vi "SensorLabview.vi"() -> ()   [LabVIEW 2020]
panel:
  in  "Water Pipe Ready":bool
  in  "Plant Health":string
  in  "Weed Detected":string
  out "VISA Error":string
  out "Return Count":dbl
  out "Website Status":string
  out "Command Status":string
  out "Pump Done Message":string
  out "Pump Command":string
  out "PumpCode":dbl
  out "Pump Duration":dbl
  out "Humidity Snapshot":dbl
  out "Temperature Snapshot":dbl
  out "Moisture %":dbl
  out "Current Pot Number":dbl
  out "Live Temperature °C":dbl
  out "Live Humidity %":dbl
  out "Selected Moisture %":dbl
  out "Humidity Voltage":dbl
  out "LM35 Voltage":dbl
  out "Selected Soil Voltage":dbl
  in  "Number of Pots":dbl
  in  "Max Pump Time":dbl
  in  "K Value":dbl
  in  "Target Moisture":dbl
  in  "Hhigh":dbl
  in  "Hlow":dbl
  in  "Vwet":dbl
  in  "Vdry":dbl
  in  "stop":bool
  in  "Robot Stop Detected":bool
  in  "ESP32 COM Port":refnum<visa-resource-name>
  # "Live Sensor Indicators"
  # "Calibration controls"
  # "System Controls"
  # "Pot snapshot indicators"
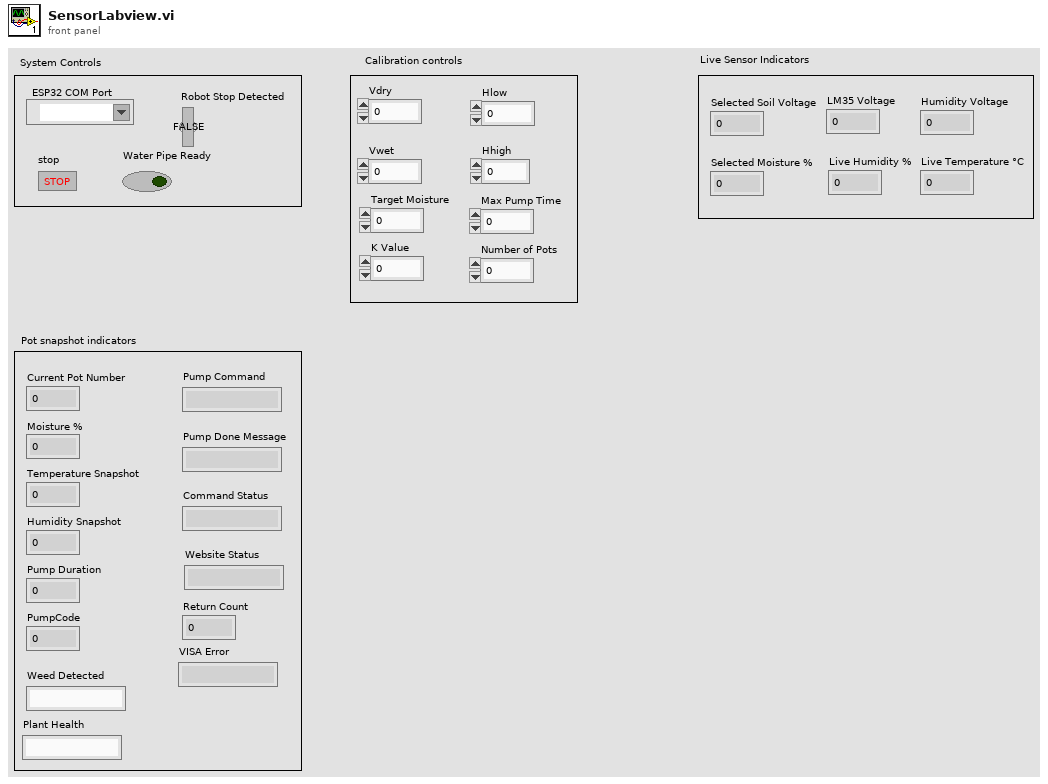
[diagram p1: front panel]
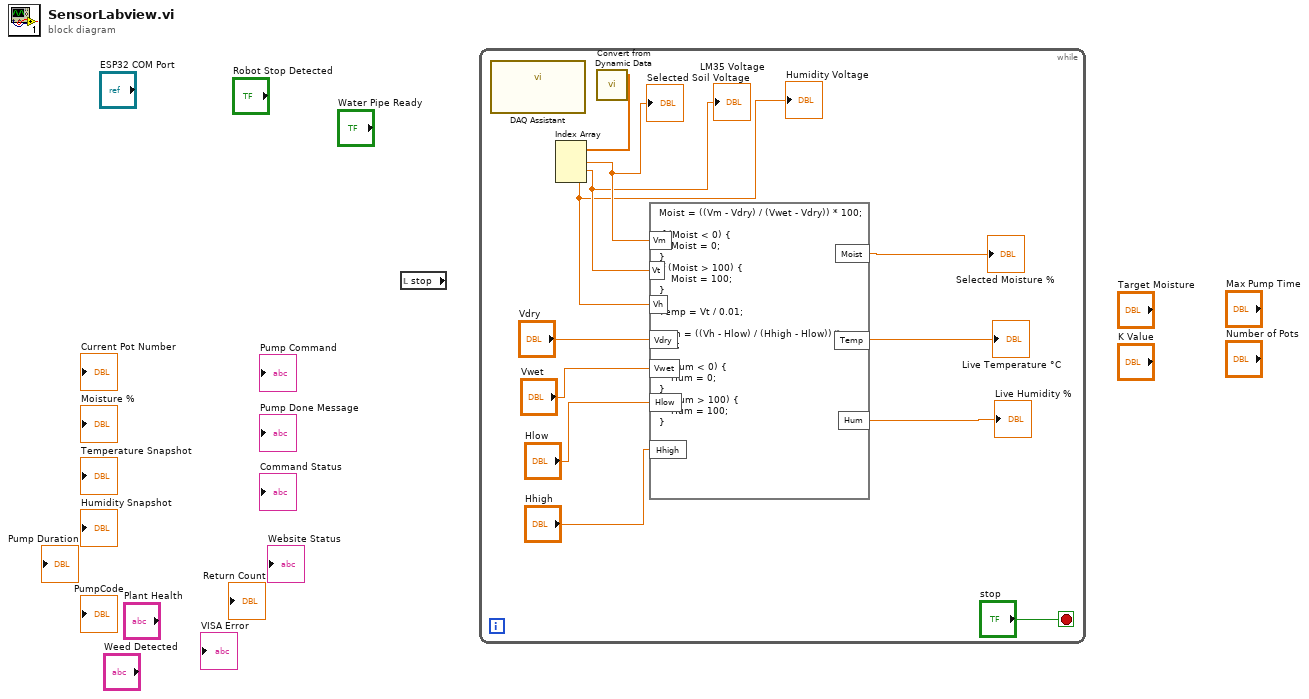
[diagram p0: block diagram]
diagram:
  n1 = local read "stop"() -> ()  [unwired: 1 out]
  n2 = while {
    stop <- "stop" stop-if-true
    n3 = call "DAQ Assistant"() -> ()  [unwired: 12 in]
    n4 = call "Convert from Dynamic Data"() -> ("Array"=w12:dbl[])  [unwired: 4 in]
    n5 = Index Array(array=w12) -> (element #1=w3:dbl, element #2=w2:dbl, element #3=w1:dbl)  [unwired: 3 in]
    "Humidity Voltage" <- w1
    "LM35 Voltage" <- w2
    "Selected Soil Voltage" <- w3
    n6 = formula code="Moist = ((Vm - Vdry) / (Vwet - Vdry)) * 100;\n\nif (Moist < 0) {\n    Moist = 0;\n}\nif (Moist > 100) {\n    Moist = 100;\n}\n\nTemp = Vt / 0.01;\n\nHum = ((Vh - Hlow) / (Hhigh - Hlow)) * 100;\n\nif (Hum < 0) {\n    Hum = 0;\n}\nif (Hum > 100) {\n    Hum = 100;\n}"("Vm"=w3, "Vt"=w2, "Vh"=w1, "Vdry"="Vdry", "Hlow"="Hlow", "Hhigh"="Hhigh", "Vwet"="Vwet") -> ("Temp"=→"Live Temperature °C":dbl, "Hum"=→"Live Humidity %":dbl, "Moist"=→"Selected Moisture %":dbl)
  }
